vi "Configure Frame.vi"(0 "VISA resource name":refnum<visa-resource-name>, 5 "Synchronized Signal Source (0:External Input)":i32(ring) items=["External Input", "Free Run", "Wide IF Video"], 7 "Frame Trigger (0.01Sec)":dbl=0.01 min=1e-06 max=1.0 format="%.6f", 9 "Frame Offset Time (0Sec)":dbl min=0.0 max=1.0 format="%.6f", 11 "error in (no error)":errorcluster) -> (4 "VISA resource name out":refnum<visa-resource-name>, 15 "error out":errorcluster)   [LabVIEW 2020, in "Anritsu Signal Analyzer Series.lvlib"]
doc: "Configures the frame settings of the spectrum analyzer."
uses:
  Anritsu Signal Analyzer Series.lvlib
panel:
  # "Sec"
  # "Sec"
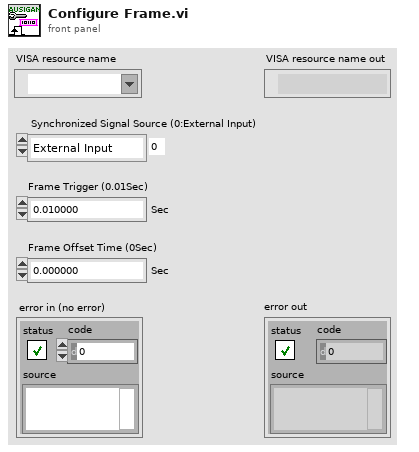
[diagram p1: front panel]
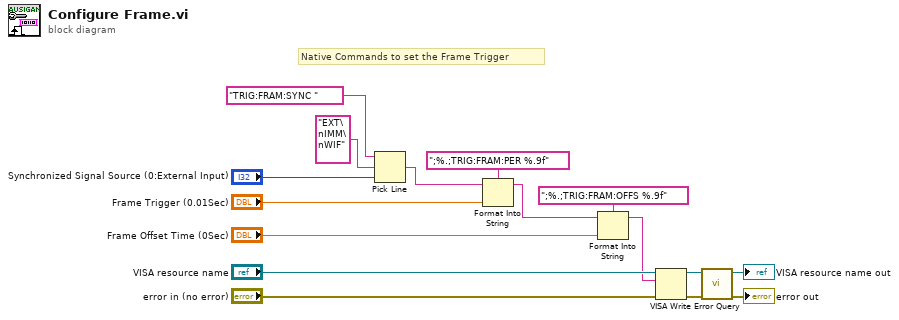
[diagram p0: block diagram]
diagram:
  # "Native Commands to set the Frame Trigger"
  n1 = Pick Line(string ("")="TRIG:FRAM:SYNC ", multi-line string="EXT\nIMM\nWIF", line index="Synchronized Signal Source (0:External Input)") -> (output string=w1:string)
  n2 = Format Into String(format string=";%.;TRIG:FRAM:PER %.9f" ("Format String"), initial string=w1, "Frame Trigger (0.01Sec)") -> (resulting string=w2:string)  [unwired: 1 in, 1 out]
  n3 = Format Into String(format string=";%.;TRIG:FRAM:OFFS %.9f" ("Format String"), initial string=w2, "Frame Offset Time (0Sec)") -> (resulting string=w3:string)  [unwired: 1 in, 1 out]
  n4 = VISA Write(VISA resource name="VISA resource name", write buffer=w3, error in (no error)="error in (no error)") -> (VISA resource name out=w11:refnum<visa-resource-name>, error out=w12:errorcluster)  [unwired: 1 out]
  n5 = call "Error Query.vi"("error in (no error)"=w12, "VISA resource name"=w11) -> ("error out"=→"error out":errorcluster, "VISA resource name out"=→"VISA resource name out":refnum<visa-resource-name>)  [unwired: 6 in, 2 out]
